vi "BRig_dataLC_Reward_OnOff_l1.vi"() -> (2 "output_Reward_OnOff":i32)   [LabVIEW 2014]
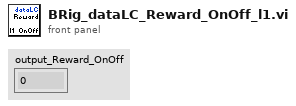
[diagram p1: front panel]
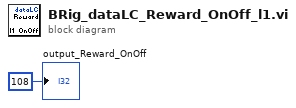
[diagram p0: block diagram]
diagram:
  "output_Reward_OnOff" <- 108 ("output_iBlock")
